vi "Publish.vi"(0 "WAMP Client in":refnum<class "WAMP Client.lvclass">, 5 "error in (no error)":errorcluster, 7 "Topic URI":string, 9 "Arguments":variant[](array[variant]), 11 "JSON Object Payload":string) -> (4 "WAMP Client out":refnum<class "WAMP Client.lvclass">, 6 "error out":errorcluster)   [LabVIEW 2020, in "WAMP Client.lvclass"]
uses:
  <userlib>/lvwamp/WAMP Client/WAMP Client.lvclass
  <userlib>/lvwamp/MessageCodes.ctl
  <userlib>/lvwamp/WAMP Client/WAMP Client.lvclass/WAMP Client.ctl
  <userlib>/lvwamp/WAMP Client/Accessors/Read Publish  Request ID Counter.vi
  <userlib>/lvwamp/WAMP Client/Accessors/Write Publish  Request ID Counter.vi
  <userlib>/lvwamp/WAMP Client/Accessors/Read Write Queue.vi
  <vilib>/JDP Science/JSONtext/JSONtext.lvlib
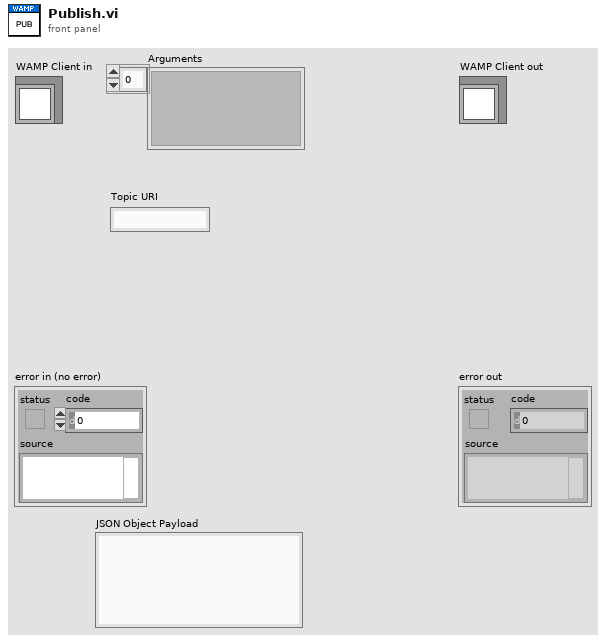
[diagram p1: front panel]
types:
  T1 = typedef "WAMP Client.lvclass/MessageCodes.ctl" = u16
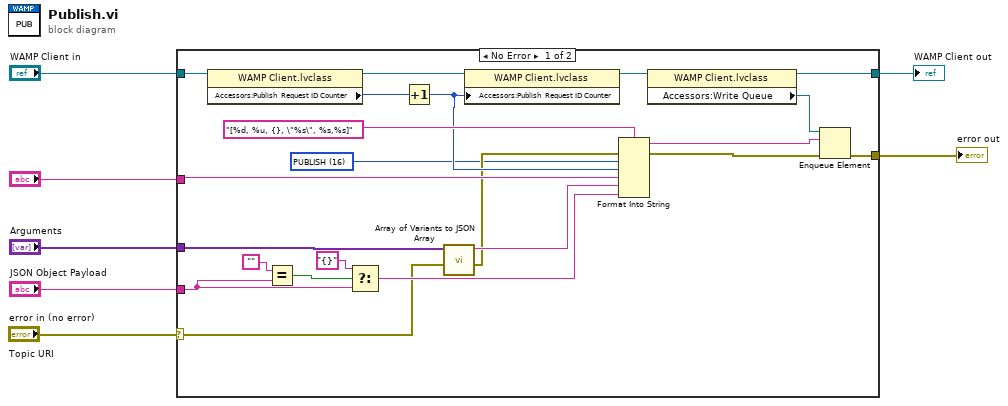
[diagram p0: block diagram]
diagram:
  n1 = case shown="No Error" "error in (no error)" {
    selector: "error in (no error)" -> [w11 w31]
    tunnel: [w29 w31] -> w6
    tunnel: [w9 w30] -> w4
    tunnel: "WAMP Client in" -> [w20 w30]
    tunnel: "Topic URI" -> [w16 _]
    tunnel: "Arguments" -> [w26 _]
    tunnel: "JSON Object Payload" -> [w22 _]
    frame No Error {
      w8 = T1 16 items=["HELLO"=1, "WELCOME"=2, "ABORT"=3, "GOODBYE"=6, "ERROR"=8, "PUBLISH"=16, "PUBLISHED"=17, "SUBSCRIBE"=32, "SUBSCRIBED"=33, "UNSUBSCRIBE"=34, "UNSUBSCRIBED"=35, "EVENT"=36, "CALL"=48, "RESULT"=59, "REGISTER"=64, "REGISTERED"=65, "UNREGISTER"=66, "UNREGISTERED"=67, "INVOCATION"=68, "YIELD"=70] ("Message Codes")
      n2 = property class="WAMP Client.lvclass"(reference=w20) -> (reference out=w15:refnum<class "WAMP Client.lvclass">, "Accessors:Publish  Request ID Counter"=w19:u32)  [unwired: 1 in, 1 out]
      n3 = Equal?(x="", y=w22) -> (x = y?=w24:bool)
      n4 = Select(t="{}", s=w24, f=w22) -> (s? t:f=w18:string)
      n5 = Increment(x=w19) -> (x+1=w14:u32)
      n6 = call <vilib>:"Array of Variants to JSON Array.vi"("error in (no error)"=w11, "Array of Variants"=w26) -> ("error out"=w10:errorcluster, "<JSON>"=w17:string)  [unwired: 8 in]
      n7 = property class="WAMP Client.lvclass"(reference=w15, "Accessors:Publish  Request ID Counter"=w14) -> (reference out=w13:refnum<class "WAMP Client.lvclass">)  [unwired: 1 in, 1 out]
      n8 = Format Into String(format string="[%d, %u, {}, \"%s\", %s,%s]" ("element"), error in=w10, w8, w14, w16, w17, w18) -> (resulting string=w27:string, error out=w25:errorcluster)  [unwired: 1 in]
      n9 = property class="WAMP Client.lvclass"(reference=w13) -> (reference out=w9:refnum<class "WAMP Client.lvclass">, "Accessors:Write Queue"=w12:refnum<queue>)  [unwired: 1 in, 1 out]
      n10 = Enqueue Element(queue=w12, element=w27, error in (no error)=w25) -> (error out=w29:errorcluster)  [unwired: 1 in, 2 out]
    }
    frame Error {
    }
  }
  "error out" <- w6
  "WAMP Client out" <- w4
